vi "Output_trigger.vi"(8 "error in (no error)":errorcluster, 11 "build_waveform in":refnum<class "build_waveform.lvclass">) -> (0 "error out":errorcluster, 2 "Array":i8[](array[numeric]), 3 "build_waveform out":refnum<class "build_waveform.lvclass">)   [LabVIEW 2019, in "build_waveform.lvclass"]
uses:
  build_waveform.lvclass
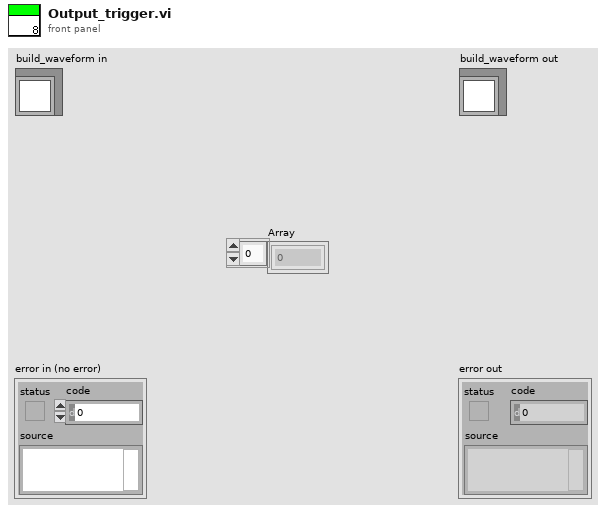
[diagram p1: front panel]
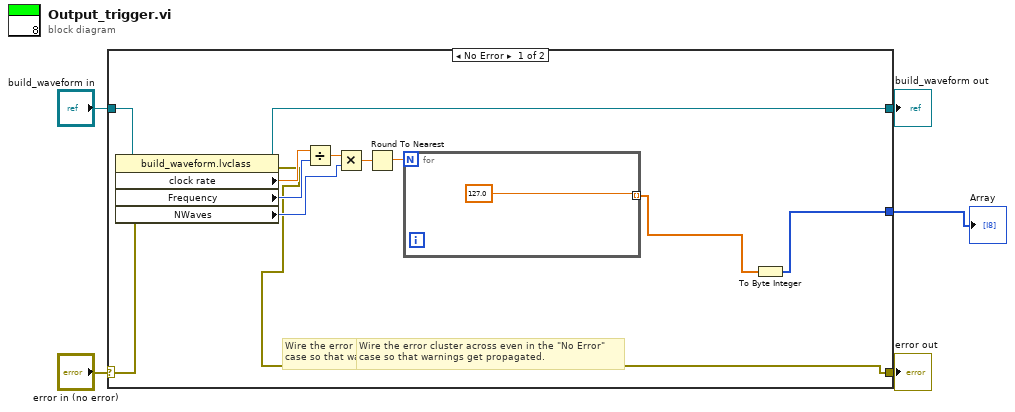
[diagram p0: block diagram]
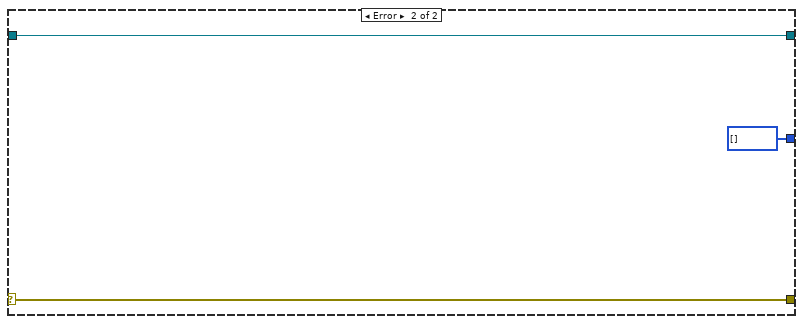
[diagram p2: hidden frame]
diagram:
  n1 = case shown="No Error" "error in (no error)" {
    selector: "error in (no error)" -> [w10 w21]
    tunnel: [w8 w21] -> w4
    tunnel: [w9 w20] -> w2
    tunnel: "build_waveform in" -> [w11 w20]
    tunnel: [w6 i8[] []] -> w1
    frame No Error {
      # "Wire the error cluster across even in the \"No Error\"\ncase so that warnings get propagated."
      # "Wire the error cluster across even in the \"No Error\"\ncase so that warnings get propagated."
      n2 = property class="build_waveform.lvclass"(reference=w11, error in=w10) -> (reference out=w9:refnum<class "build_waveform.lvclass">, error out=w8:errorcluster, "clock rate"=w17:dbl, "Frequency"=w12:i32, "NWaves"=w16:i32)
      n3 = Divide(x=w17, y=w12) -> (x/y=w15:dbl)
      n4 = Multiply(x=w15, y=w16) -> (x*y=w14:dbl)
      n5 = Round To Nearest(number=w14) -> (nearest integer value=w13:dbl)
      n6 = for {
        N: w13 -> [_]
        tunnel: [127.0 ("y")] -> w7 mode=indexing
      }
      n7 = To Byte Integer(number=w7) -> (8bit integer=w6:i8[])
    }
    frame Error {
    }
  }
  "error out" <- w4
  "build_waveform out" <- w2
  "Array" <- w1
